vi "PQgetlength.vi"(7 "error in (no error)":errorcluster, 8 "field_num":i32, 9 "tup_num":i32, 10 "res":u32) -> (0 "error out":errorcluster, 2 "length":u32, 3 "res_out":u32)   [LabVIEW 2019, in "libpqlv.lvlib"]
doc: "Returns the actual length of a field value in bytes. Row and column numbers start at 0.\nThis is the actual data length for the particular data value, that is, the size of the object pointed to by PQgetvalue. For text data format this is the same as strlen(). For binary format this is essential information. Note that one should not rely on PQfsize to obtain the actual data length."
uses:
  libpqlv.lvlib
  libpq.dll
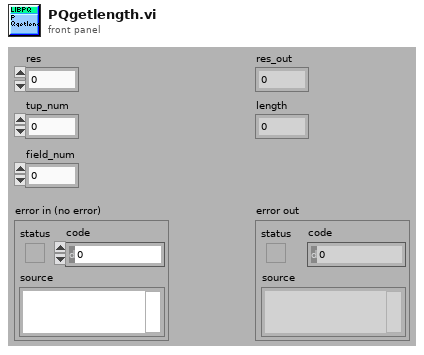
[diagram p1: front panel]
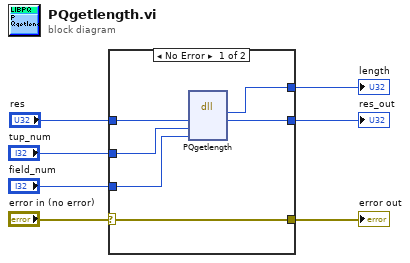
[diagram p0: block diagram]
diagram:
  n1 = case shown="No Error" "error in (no error)" {
    selector: "error in (no error)" -> [w13 w15]
    tunnel: [w13 w15] -> w6
    tunnel: [w12 _] -> w5
    tunnel: "tup_num" -> [w11 _]
    tunnel: "field_num" -> [w10 _]
    tunnel: [w9 w14] -> w2
    tunnel: "res" -> [w8 w14]
    frame No Error {
      n2 = dll-call lib="libpq.*" fn="PQgetlength"("res"=w8, "tup_num"=w11, "field_num"=w10) -> ("length"=w12:u32, "res"=w9:u32)  [unwired: 5 in, 2 out]
    }
    frame Error {
    }
  }
  "length" <- w5
  "error out" <- w6
  "res_out" <- w2
